vi "散斑模块.vi"(1 "散斑类型":u16(ring) items=["随机散斑", "未定"], 2 "采样次数":i32, 3 "光源行数":i32) -> (0 "输出簇":T1)   [LabVIEW 2018]
uses:
  <vilib>/imath/engines/lvmath2/RunTimeEngine/BuiltInFunctions/rand/NIMS_rand(1,I32).vi
  <vilib>/imath/engines/lvmath2/RunTimeEngine/ErrorHandling/NIMS_Error From Error Code.vi
  <vilib>/imath/engines/lvmath2/RunTimeEngine/BuiltInFunctions/sum/NIMS_sum(GV).vi
  <instcachedir>/0/NIMS_sum(GV)_67F5EC36BC034E54A6BEC5B0673C00E5.lvgen/NIMS_sum(GV)_67F5EC36BC034E54A6BEC5B0673C00E5_000.vi
  <vilib>/imath/engines/lvmath2/RunTimeEngine/NodeEndStatement/NIMS_NodeEndStatement_Output.vi
  <instcachedir>/0/NIMS_NodeEndStatement_Output_53EC0D466D134D7ABD903AC30B43404B.lvgen/NIMS_NodeEndStatement_Output_53EC0D466D134D7ABD903AC30B43404B_005.vi
  <vilib>/imath/engines/lvmath2/RunTimeEngine/ErrorHandling/NIMS_Finalize Error.vi
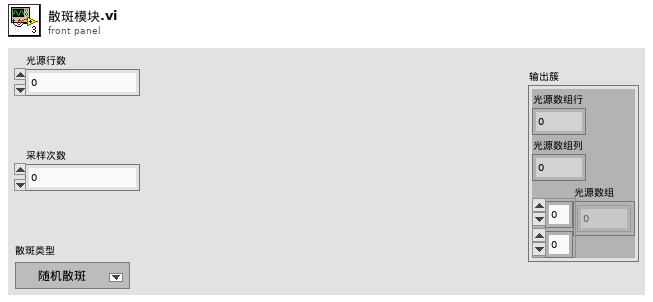
[diagram p1: front panel]
types:
  T1 = cluster{"光源数组行":i32, "光源数组列":i32, "光源数组":dbl[][]}
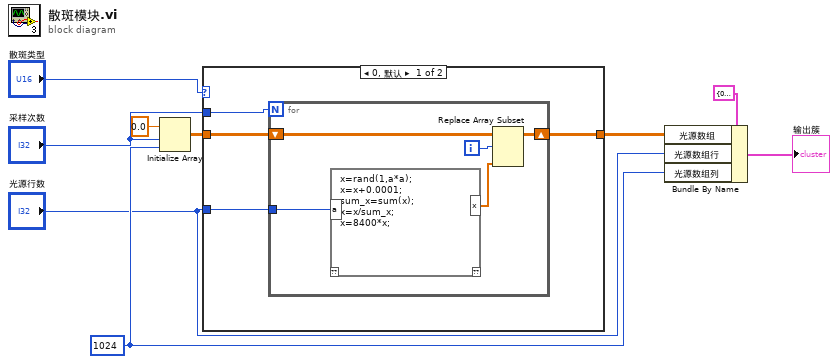
[diagram p0: block diagram]
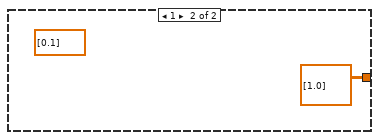
[diagram p2: hidden frame]
diagram:
  w7 = 1024
  n1 = Initialize Array(0.0, "采样次数", w7) -> (w3:dbl[][])
  n2 = case shown="0, 默认" "散斑类型" {
    tunnel: "采样次数" -> [w13 _]
    tunnel: w3 -> [w12 _]
    tunnel: "光源行数" -> [w11 _]
    tunnel: [w10 dbl[][] [[1.0]]] -> w1
    frame 0, Default {
      n3 = for {
        N: w13 -> [_]
        shift-right: [w16] -> w10
        shift-left: w12 -> [w18]
        tunnel: w11 -> [w15]
        i -> [w17]
        n4 = mathscript code="x=rand(1,a*a);\nx=x+0.0001;\nsum_x=sum(x);\nx=x/sum_x;\nx=8400*x;"("a"=w15) -> ("x"=w14:dbl[])  [unwired: 1 in, 1 out]
        n5 = Replace Array Subset(array=w18, new element=w14, index (row)=w17) -> (w16:dbl[][])  [unwired: 1 in]
      }
    }
    frame 1 {
      (unwired) dbl[] [0.1] ("数组")
    }
  }
  n6 = Bundle By Name(cluster=T1 {"光源数组行"=0, "光源数组列"=0, "光源数组"=[]}, "光源数组"=w1, "光源数组行"="光源行数", "光源数组列"=w7) -> (→"输出簇":T1)
